vi "Biometry Ascan Parameter2String.vi"(8 "error in (no error)":errorcluster caption="错误输入（无错误）", 9 "Biometry Parameter":T2, 10 "Biometry State":T1, 11 "No":i32) -> (0 "error out":errorcluster caption="错误输出", 2 "Data Output":string[](array[string]))   [LabVIEW 2015, in "Utility VIs.lvlib"]
doc: "该模板用于创建子VI。"
uses:
  Utility VIs.lvlib
  Database Processing/Support/Table/Biometry Parameter.ctl
  Database Processing/Support/Table/Biometry State.ctl
  Database Processing/Database Processing.lvlib
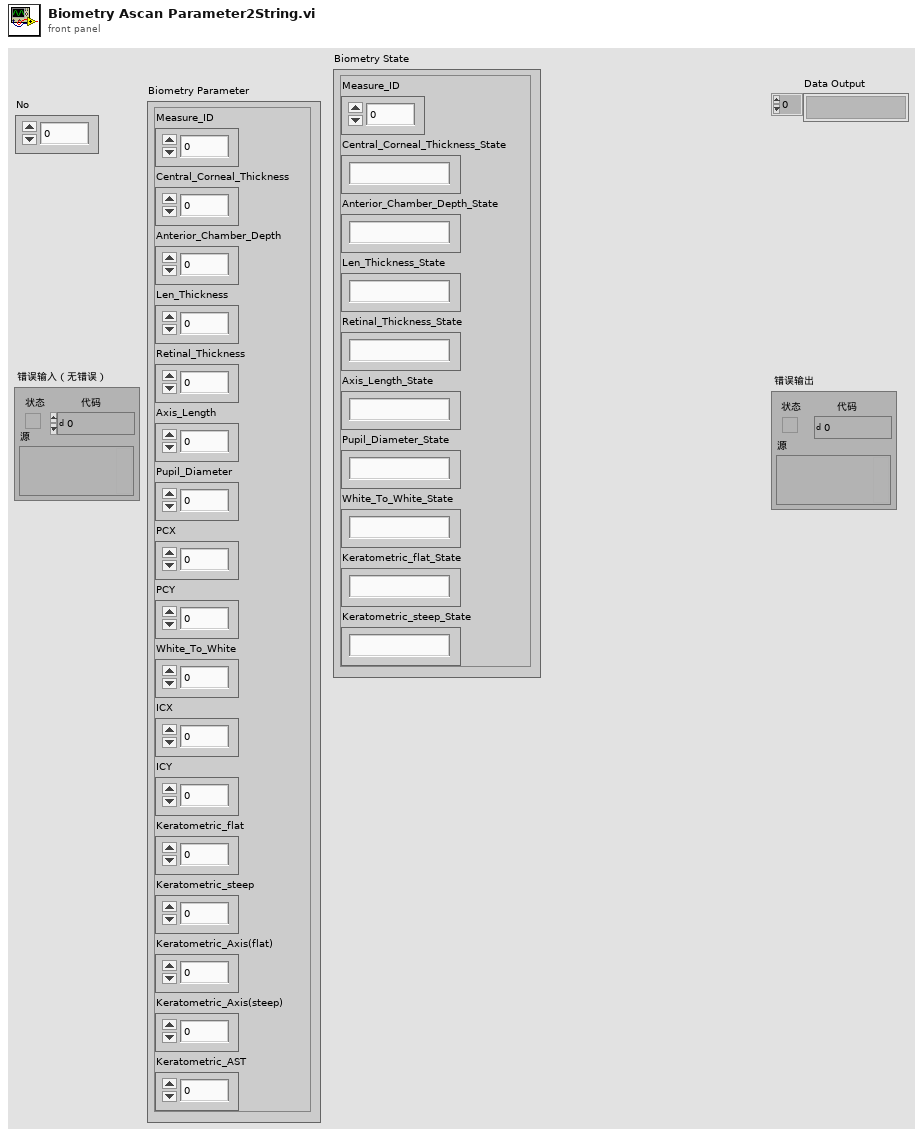
[diagram p1: front panel]
types:
  T1 = typedef "Database Processing.lvlib/Biometry State.ctl" = cluster{"Measure_ID":i64, "Central_Corneal_Thickness_State":string, "Anterior_Chamber_Depth_State":string, "Len_Thickness_State":string, "Retinal_Thickness_State":string, "Axis_Length_State":string, "Pupil_Diameter_State":string, "White_To_White_State":string, "Keratometric_flat_State":string, "Keratometric_steep_State":string}
  T2 = typedef "Database Processing.lvlib/Biometry Parameter.ctl" = cluster{"Measure_ID":i64, "Central_Corneal_Thickness":sgl, "Anterior_Chamber_Depth":sgl, "Len_Thickness":sgl, "Retinal_Thickness":sgl, "Axis_Length":sgl, "Pupil_Diameter":sgl, "PCX":sgl, "PCY":sgl, "White_To_White":sgl, "ICX":sgl, "ICY":sgl, "Keratometric_flat":sgl, "Keratometric_steep":sgl, "Keratometric_Axis(flat)":sgl, "Keratometric_Axis(steep)":sgl, "Keratometric_AST":sgl}
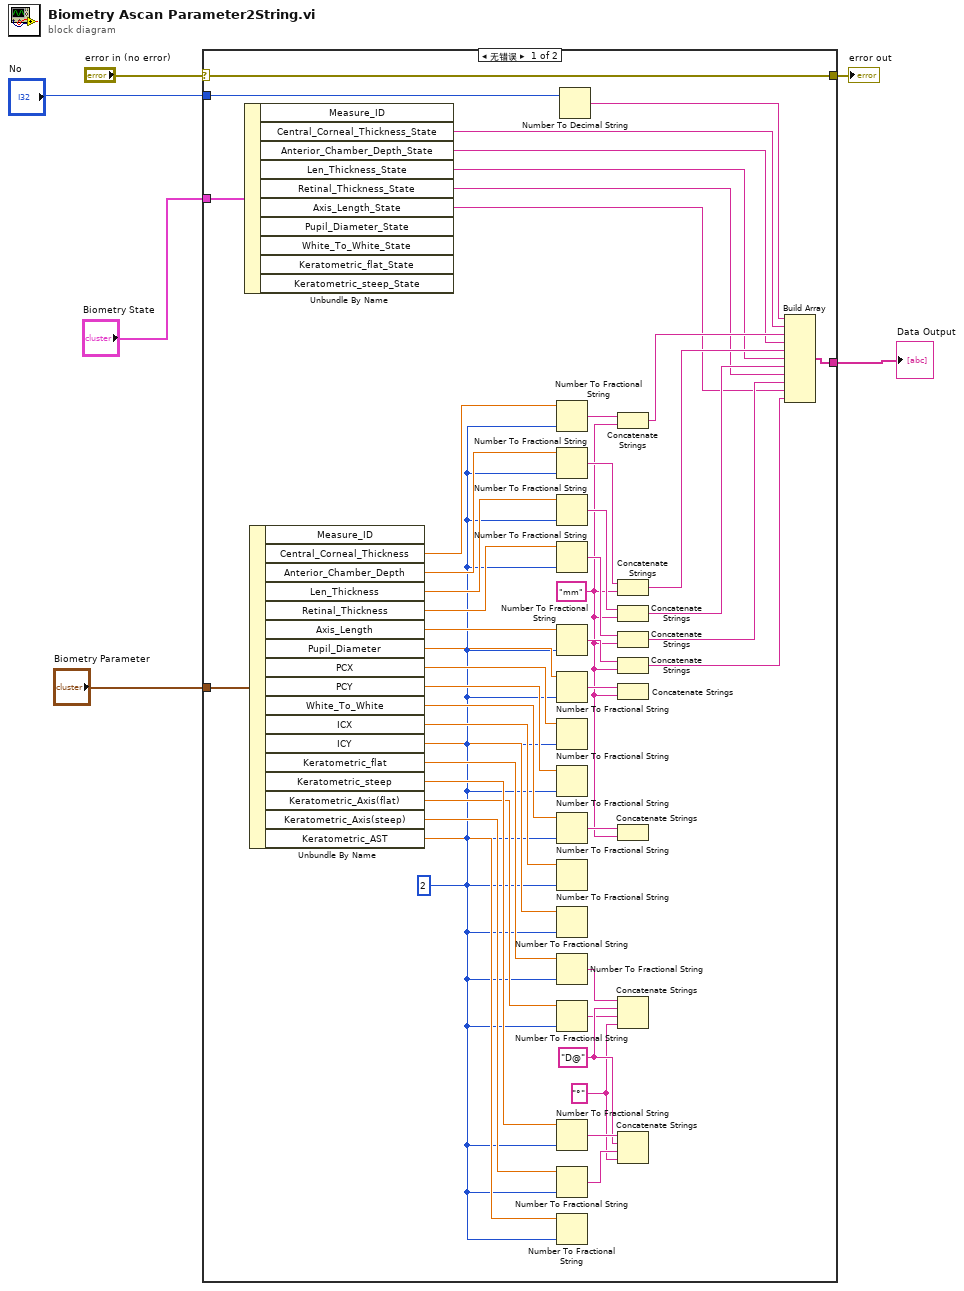
[diagram p0: block diagram]
diagram:
  n1 = case shown="无错误" "error in (no error)" {
    selector: "error in (no error)" -> [w20 w54]
    tunnel: [w20 w54] -> w5
    tunnel: "Biometry Parameter" -> [w53 _]
    tunnel: "Biometry State" -> [w52 _]
    tunnel: [w9 _] -> w2
    tunnel: "No" -> [w8 _]
    frame No Error {
      w21 = "°" ("字符串")
      w27 = "D@" ("字符串")
      w28 = "mm" ("字符串")
      w23 = i16 2 ("精度(6)")
      n2 = Unbundle By Name(w52) -> ("Central_Corneal_Thickness_State"=w14:string, "Anterior_Chamber_Depth_State"=w13:string, "Len_Thickness_State"=w12:string, "Retinal_Thickness_State"=w11:string, "Axis_Length_State"=w10:string)  [unwired: 5 out]
      n3 = Unbundle By Name(w53) -> ("Central_Corneal_Thickness"=w51:sgl, "Anterior_Chamber_Depth"=w50:sgl, "Len_Thickness"=w49:sgl, "Retinal_Thickness"=w48:sgl, "Axis_Length"=w47:sgl, "Pupil_Diameter"=w46:sgl, "PCX"=w45:sgl, "PCY"=w44:sgl, "White_To_White"=w43:sgl, "ICX"=w42:sgl, "ICY"=w41:sgl, "Keratometric_flat"=w40:sgl, "Keratometric_steep"=w39:sgl, "Keratometric_Axis(flat)"=w38:sgl, "Keratometric_Axis(steep)"=w25:sgl, "Keratometric_AST"=w24:sgl)  [unwired: 1 out]
      n4 = Number To Fractional String(number=w51, precision (6)=w23) -> (F-format string=w37:string)  [unwired: 2 in]
      n5 = Number To Fractional String(number=w50, precision (6)=w23) -> (F-format string=w36:string)  [unwired: 2 in]
      n6 = Number To Fractional String(number=w49, precision (6)=w23) -> (F-format string=w35:string)  [unwired: 2 in]
      n7 = Number To Fractional String(number=w48, precision (6)=w23) -> (F-format string=w34:string)  [unwired: 2 in]
      n8 = Number To Fractional String(number=w47, precision (6)=w23) -> (F-format string=w33:string)  [unwired: 2 in]
      n9 = Number To Fractional String(number=w46, precision (6)=w23) -> (F-format string=w32:string)  [unwired: 2 in]
      n10 = Number To Fractional String(number=w45, precision (6)=w23) -> ()  [unwired: 2 in, 1 out]
      n11 = Number To Fractional String(number=w44, precision (6)=w23) -> ()  [unwired: 2 in, 1 out]
      n12 = Number To Fractional String(number=w43, precision (6)=w23) -> (F-format string=w31:string)  [unwired: 2 in]
      n13 = Number To Fractional String(number=w42, precision (6)=w23) -> ()  [unwired: 2 in, 1 out]
      n14 = Number To Fractional String(number=w41, precision (6)=w23) -> ()  [unwired: 2 in, 1 out]
      n15 = Number To Fractional String(number=w40, precision (6)=w23) -> (F-format string=w30:string)  [unwired: 2 in]
      n16 = Number To Fractional String(number=w38, precision (6)=w23) -> (F-format string=w26:string)  [unwired: 2 in]
      n17 = Number To Fractional String(number=w39, precision (6)=w23) -> (F-format string=w29:string)  [unwired: 2 in]
      n18 = Number To Fractional String(number=w25, precision (6)=w23) -> (F-format string=w22:string)  [unwired: 2 in]
      n19 = Number To Fractional String(number=w24, precision (6)=w23) -> ()  [unwired: 2 in, 1 out]
      n20 = Number To Decimal String(number=w8) -> (decimal integer string=w7:string)  [unwired: 1 in]
      n21 = Concatenate Strings(w37, w28) -> (w19:string)
      n22 = Concatenate Strings(w36, w28) -> (w18:string)
      n23 = Concatenate Strings(w35, w28) -> (w17:string)
      n24 = Concatenate Strings(w34, w28) -> (w16:string)
      n25 = Concatenate Strings(w33, w28) -> (w15:string)
      n26 = Concatenate Strings(w32, w28) -> ()  [unwired: 1 out]
      n27 = Concatenate Strings(w31, w28) -> ()  [unwired: 1 out]
      n28 = Concatenate Strings(w30, w27, w26, w21) -> ()  [unwired: 1 out]
      n29 = Concatenate Strings(w29, w27, w22, w21) -> ()  [unwired: 1 out]
      n30 = Build Array(w7, w14, w19, w13, w18, w12, w17, w11, w16, w10, w15) -> (w9:string[])
    }
    frame Error {
    }
  }
  "error out" <- w5
  "Data Output" <- w2
